vi "Read Refnum Table.vi"(11 "Typed Refnum Table In":variant) -> (2 "Refnum Groups":T1(array[cluster]))   [LabVIEW 2015, in "ActorEvents.lvlib" / "ActorAutoRegistration.lvclass"]
uses:
  ActorAutoRegistration.lvclass
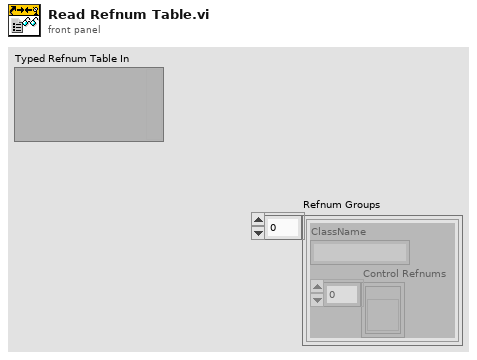
[diagram p1: front panel]
types:
  T1 = cluster{"ClassName":string, "Control Refnums":refnum<vi>[]}[]
  T2 = cluster{"ClassName":string, "Control Refnums":refnum<vi>[]}
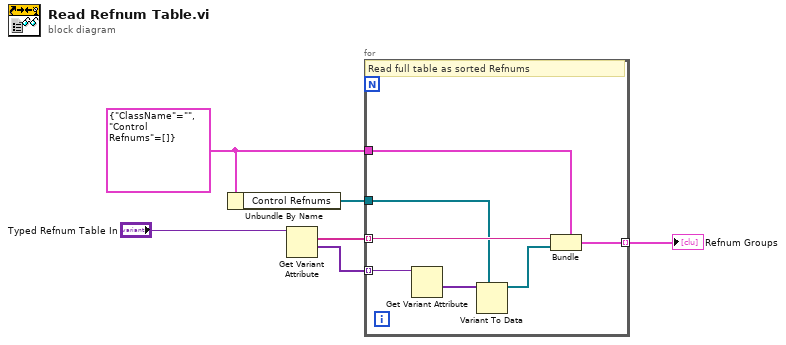
[diagram p0: block diagram]
diagram:
  w2 = T2 {"ClassName"="", "Control Refnums"=[]} ("Refnum Group")
  n1 = Unbundle By Name(w2) -> ("Control Refnums"=w1:refnum<vi>[])
  n2 = Get Variant Attribute(Variant="Typed Refnum Table In") -> (names=w4:string[], values=w5:variant[])  [unwired: 3 in, 2 out]
  n3 = for {
    tunnel: w5 -> [w13] mode=indexing
    tunnel: w4 -> [w11] mode=indexing
    tunnel: w2 -> [w12]
    tunnel: [w10] -> w3 mode=indexing
    tunnel: w1 -> [w9]
    # "Read full table as sorted Refnums"
    n4 = Get Variant Attribute(Variant=w13) -> (values=w8:variant[])  [unwired: 3 in, 3 out]
    n5 = Variant To Data(type=w9, Variant=w8) -> (data=w7:refnum<vi>[])  [unwired: 1 in, 1 out]
    n6 = Bundle(cluster=w12, "ClassName"=w11, "Control Refnums"=w7) -> (w10:T2)
  }
  "Refnum Groups" <- w3
